vi "Smart_Traffic_Light_System_Main.vi"() -> ()   [LabVIEW 2022 SP3]
uses:
  Chamath Labview/TrafficLightStates.ctl
  <vilib>/DAQmx/read.llb/DAQmx Read (Analog 1D DBL NChan 1Samp).vi
  <vilib>/DAQmx/write.llb/DAQmx Write (Digital Bool 1Line 1Point).vi
  <vilib>/DAQmx/read.llb/DAQmx Read (Digital Bool 1Line 1Point).vi
  <vilib>/Utility/error.llb/Trim Whitespace One-Sided.vi
  <vilib>/DAQmx/create/channels.llb/DAQmx Create Channel (DO-Digital Output).vi
  <vilib>/DAQmx/create/channels.llb/DAQmx Create Channel (AI-Voltage-Basic).vi
  <vilib>/DAQmx/create/channels.llb/DAQmx Create Channel (DI-Digital Input).vi
  <vilib>/DAQmx/miscellaneous.llb/DAQmx Fill In Error Info.vi
panel:
  out "?":string
  out "Street Lights":bool
  in  "Rain signal":tag
  out "Temp 2":bool
  out "Temp 1":bool
  in  "Ped Green":tag
  in  "Ped red":tag
  in  "Numeric":dbl
  out "Square 2":dynamicdata(graph) caption="Square"
  in  "Amplitude":dbl=2.5
  in  "Offset":dbl=2.5
  in  "Frequency":dbl=50.0
  in  "stop (F)":bool
  out "Heavy Rain":bool
  out "Stop Light":bool
  out "Level 7":bool
  out "?":string
  out "Medium rain":bool
  out "Light rain":bool
  out "No rain":bool
  out "?":string
  out "Level 6":bool
  out "Level 5":bool
  out "Level 4":bool
  out "Level 3":bool
  out "Level 2":bool
  out "Level 1":bool
  out "?":string
  out "?":string
  in  "?":bool
  out "?":string
  out "?":string
  in  "Heavy Rain threshold":dbl
  in  "LDR Threshold":dbl
  in  "Buzzer 2":u16(ring) items=["DO0", "DO1", "DO4", "DO5", "DO6"]
  in  "LDR 2":u16(ring) items=["AI1", "AI2", "AI3", "AI4"]
  in  "Rain sensor":u16(ring) items=["AI1", "AI1", "AI3", "AI4"]
  out "Pedestrian in":bool
  out "Push Switch In":bool
  in  "push switch":tag
  out "Push Switch":bool
  out "Rain":bool
  in  "Rain Sensor Output Channel":tag
  in  "LDR output channel":tag
  out "LDR voltage":dbl(knob) scale=0.0..5.0
  out "Rain Sensor Voltage":dbl(knob) scale=0.0..10.0
  in  "Analog input channel":tag
  in  "buzzer - Po.0":tag
  out "Buzzer":bool
  out "RED":bool
  out "YELLOW":bool
  out "green":bool
  out "Pedestrians":bool
  in  "DAQmx Physical Channel 6":tag
  in  "DAQmx Physical Channel 5":tag
  in  "DAQmx Physical Channel 4":tag
  in  "Enum":T1
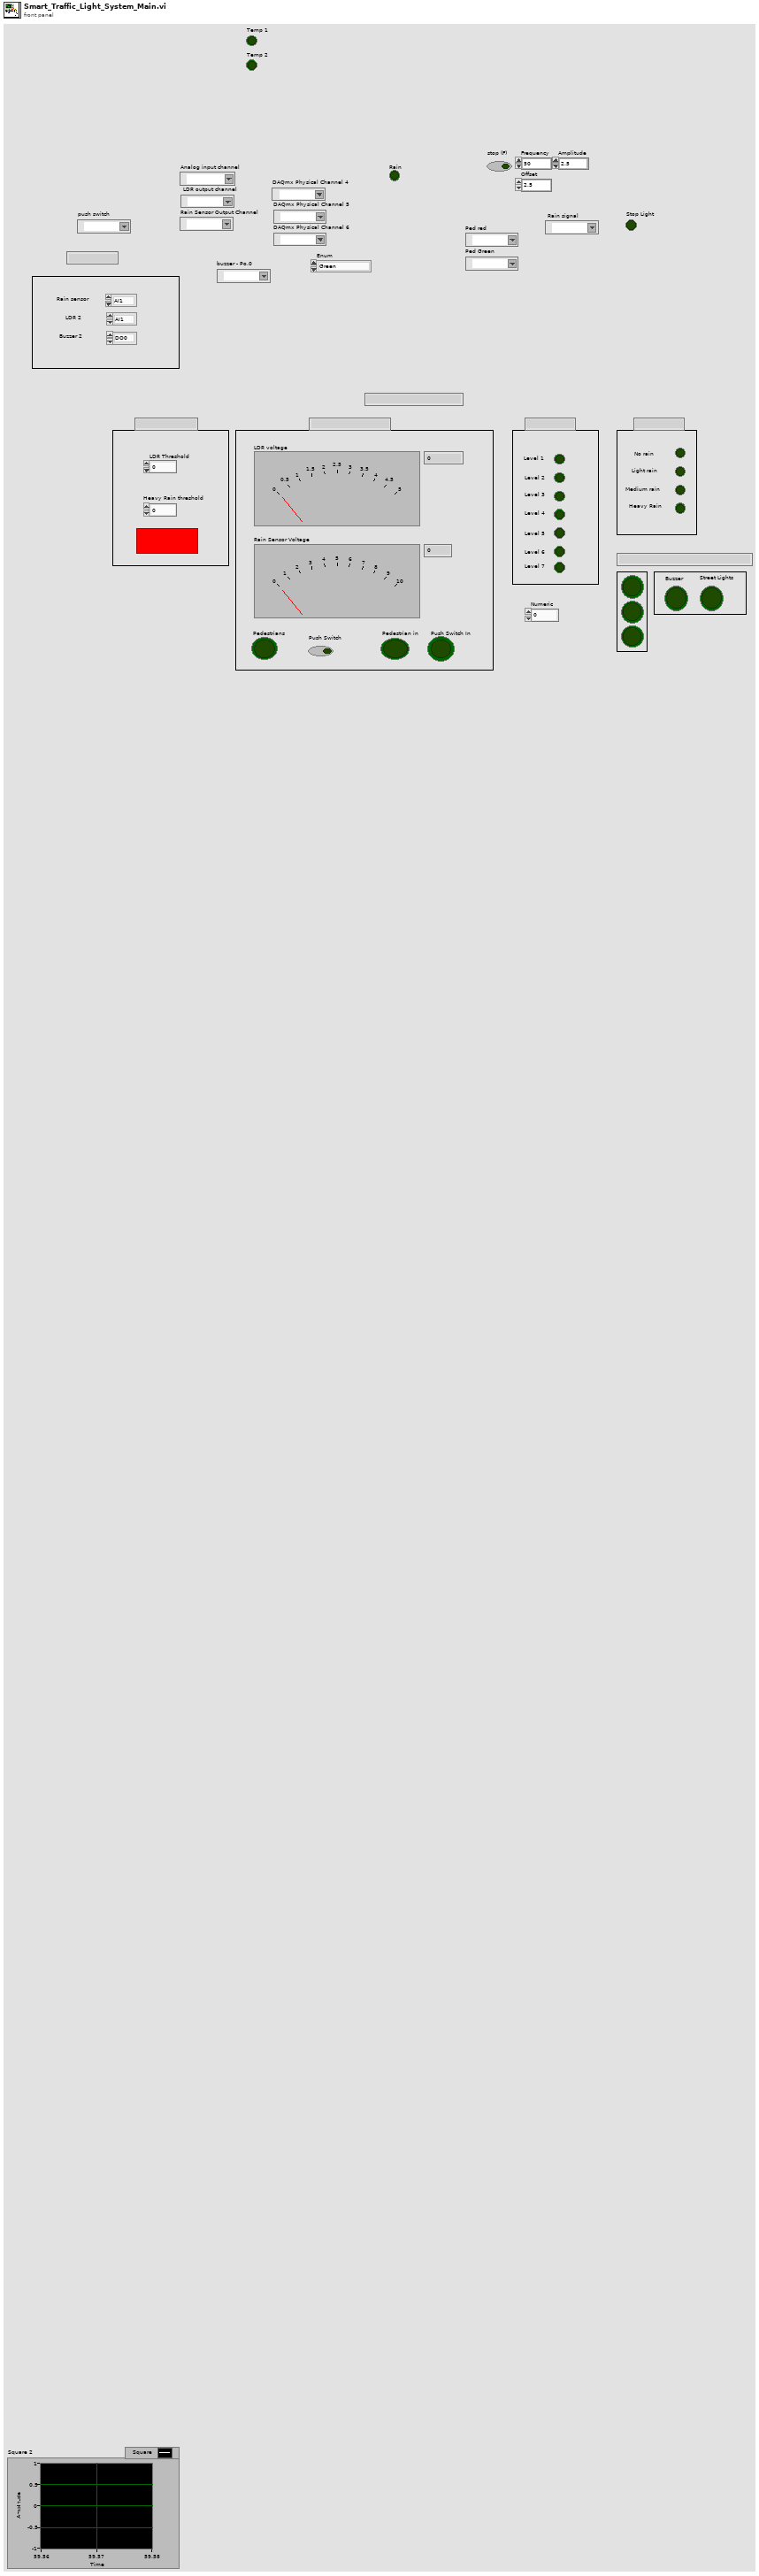
[diagram p1: front panel]
types:
  T1 = typedef "TrafficLightStates.ctl" = enum16{"Green", "Yellow1", "Red", "Yellow2"}
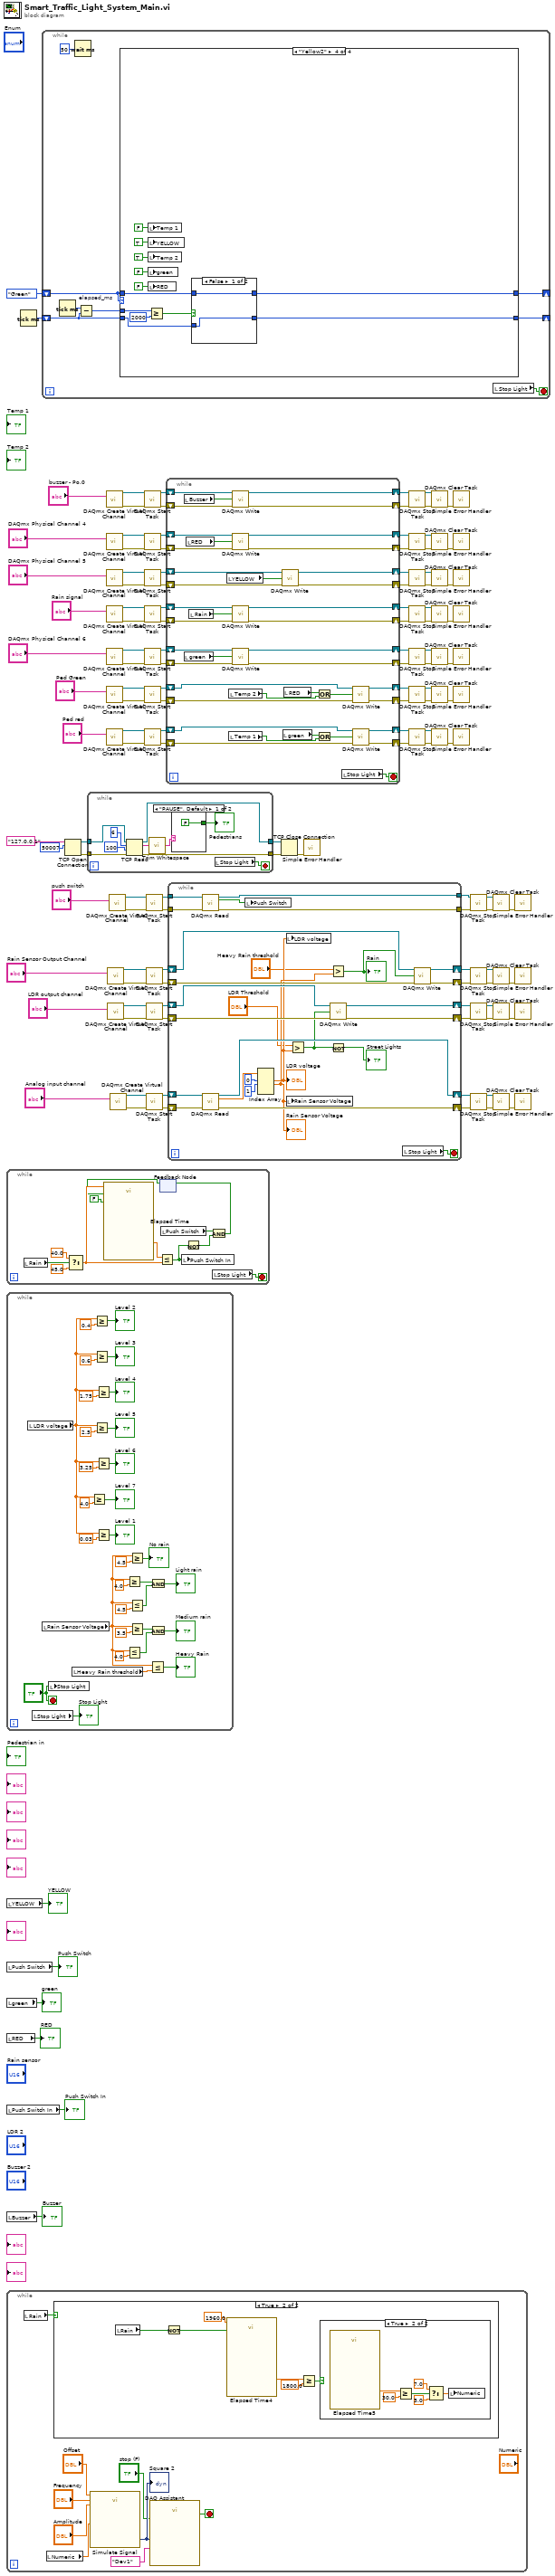
[diagram p0: block diagram]
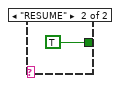
[diagram p4: hidden frame]
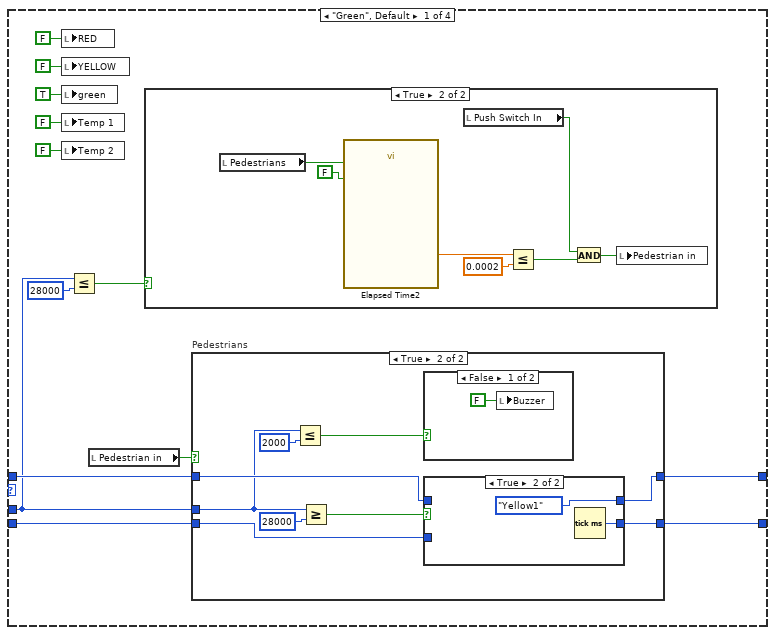
[diagram p5: hidden frame]
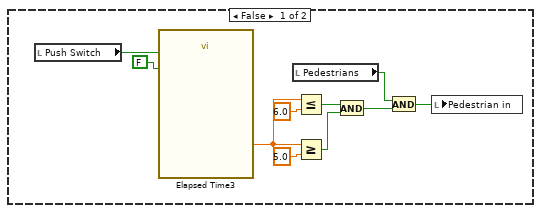
[diagram p6: hidden frame]
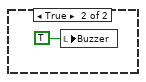
[diagram p8: hidden frame]
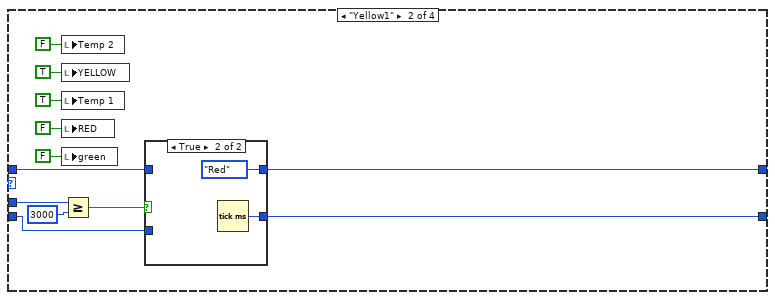
[diagram p10: hidden frame]
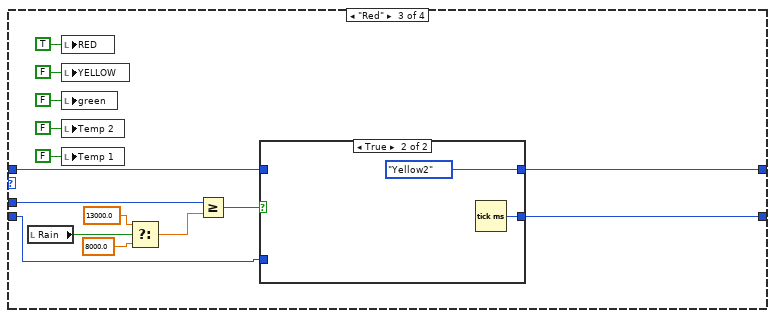
[diagram p12: hidden frame]
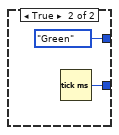
[diagram p14: hidden frame]
diagram:
  n1 = while {
    stop <- w126 stop-if-true
    n2 = local read "Rain"() -> (w135:bool)
    n3 = Select(t=40.0, s=w135, f=45.0) -> (s? t:f=w132:dbl)
    n4 = feedback #1() -> (w127:bool)  [unwired: 1 in]
    n5 = call "Elapsed Time"("Time Target (s)"=w132, "Reset"=w127, "Auto Reset"=FALSE) -> ("Elapsed Time (s)"=w136:dbl)  [unwired: 9 in, 7 out]
    n6 = Less Or Equal?(x=w136, y=w132) -> (x <= y?=w130:bool)
    n7 = local read "Push Switch"() -> (w131:bool)
    n8 = local write "Push Switch In"(w130) -> ()
    n9 = Not(x=w130) -> (.not. x?=w129:bool)
    n10 = And(x=w131, y=w129) -> (x .and. y?=w128:bool)
    n11 = feedback-in #1(w128) -> ()
    n12 = local read "Stop Light"() -> (w126:bool)
  }
  n13 = while {
    stop <- "?" stop-if-true
    n14 = local read "LDR voltage"() -> (w167:dbl)
    n15 = local read "Stop Light"() -> (→"Stop Light":bool)
    n16 = local read "Rain Sensor Voltage"() -> (w152:dbl)
    n17 = local write "Stop Light"("?") -> ()
    n18 = local read "Heavy Rain threshold"() -> (w138:dbl)
    n19 = Greater Or Equal?(x=w167, y=4.0) -> (x >= y?=→"Level 7":bool)
    n20 = Greater Or Equal?(x=w167, y=0.4) -> (x >= y?=→"Level 2":bool)
    n21 = Greater Or Equal?(x=w167, y=0.6) -> (x >= y?=→"Level 3":bool)
    n22 = Greater Or Equal?(x=w167, y=2.5) -> (x >= y?=→"Level 5":bool)
    n23 = Greater Or Equal?(x=w167, y=1.75) -> (x >= y?=→"Level 4":bool)
    n24 = Greater Or Equal?(x=w167, y=3.25) -> (x >= y?=→"Level 6":bool)
    n25 = Greater Or Equal?(x=w167, y=0.03) -> (x >= y?=→"Level 1":bool)
    n26 = Greater Or Equal?(x=w152, y=4.0) -> (x >= y?=w146:bool)
    n27 = Less Or Equal?(x=w152, y=4.0) -> (x <= y?=w143:bool)
    n28 = Greater Or Equal?(x=w152, y=4.5) -> (x >= y?=→"No rain":bool)
    n29 = Less Or Equal?(x=w152, y=4.5) -> (x <= y?=w145:bool)
    n30 = Greater Or Equal?(x=w152, y=3.5) -> (x >= y?=w144:bool)
    n31 = Less Or Equal?(x=w152, y=w138) -> (x <= y?=→"Heavy Rain":bool)
    n32 = And(x=w146, y=w145) -> (x .and. y?=→"Light rain":bool)
    n33 = And(x=w144, y=w143) -> (x .and. y?=→"Medium rain":bool)
  }
  n34 = local read "YELLOW"() -> (→"YELLOW":bool)
  n35 = local read "Push Switch"() -> (→"Push Switch":bool)
  n36 = local read "green"() -> (→"green":bool)
  n37 = local read "RED"() -> (→"RED":bool)
  n38 = local read "Push Switch In"() -> (→"Push Switch In":bool)
  n39 = local read "Buzzer"() -> (→"Buzzer":bool)
  n40 = while {
    stop <- w178 stop-if-true
    n41 = local read "Rain"() -> (w171:bool)
    n42 = local read "Numeric"() -> (w170:dbl)
    n43 = case shown="True" w171 {
      frame False {
      }
      frame True {
        n44 = local read "Rain"() -> (w183:bool)
        n45 = Not(x=w183) -> (.not. x?=w182:bool)
        n46 = call "Elapsed Time4"("Time Target (s)"=1960.0, "Reset"=w182) -> ("Elapsed Time (s)"=w181:dbl)  [unwired: 10 in, 7 out]
        n47 = Greater Or Equal?(x=w181, y=1800.0) -> (x >= y?=w179:bool)
        n48 = case shown="True" w179 {
          frame False {
          }
          frame True {
            n49 = call "Elapsed Time5"() -> ("Elapsed Time (s)"=w190:dbl)  [unwired: 12 in, 7 out]
            n50 = Greater Or Equal?(x=w190, y=30.0) -> (x >= y?=w188:bool)
            n51 = Select(t=7.0, s=w188, f=3.0) -> (s? t:f=w185:dbl)
            n52 = local write "Numeric"(w185) -> ()
          }
        }
      }
    }
    n53 = call "Simulate Signal"("Offset"="Offset", "Duty Cycle (%)"=w170, "Frequency"="Frequency", "Amplitude"="Amplitude") -> ("Square"=w177:dynamicdata)  [unwired: 10 in, 1 out]
    "Square 2" <- w177
    n54 = call "DAQ Assistant"("data"=w177, "stop (F)"="stop (F)", "device name"=tag "Dev1") -> ("stopped"=w178:bool)  [unwired: 14 in, 2 out]
  }
  n55 = Tick Count (ms)() -> (millisecond timer value=w125:u32)
  n56 = while {
    shift-right: [w196] -> _
    shift-left: TrafficLightStates."Green" ("Enum") -> [w197]
    shift-right: [w194] -> _
    shift-left: w125 -> [w195]
    stop <- w191 stop-if-true
    n57 = Tick Count (ms)() -> (millisecond timer value=w198:u32)
    n58 = Wait (ms)(milliseconds to wait=u32 50) -> ()  [unwired: 1 out]
    n59 = Subtract "elapsed_ms"(x=w198, y=w195) -> (x-y=w193:u32)
    n60 = case shown="\"Yellow2\"" w197 {
      tunnel: w197 -> [w211 w252 w271 w287]
      tunnel: [w210 w254 w272 w289] -> w196
      tunnel: w195 -> [w209 w251 w270 w286]
      tunnel: [w208 w253 w269 w288] -> w194
      tunnel: w193 -> [w204 w257 w274 w292]
      frame "Green", Default {
        n61 = local write "RED"(FALSE ("red")) -> ()
        n62 = local write "YELLOW"(FALSE ("yellow")) -> ()
        n63 = local write "green"(TRUE ("green")) -> ()
        n64 = local write "Temp 1"(FALSE ("Temp 1")) -> ()
        n65 = local write "Temp 2"(FALSE ("Temp 2")) -> ()
        n66 = Less Or Equal?(x=w204, y=u32 28000) -> (x <= y?=w202:bool)
        n67 = local read "Pedestrian in"() -> (w201:bool)
        n68 = case shown="True" w202 {
          frame False {
            n69 = local read "Push Switch"() -> (w221:bool)
            n70 = call "Elapsed Time3"("Reset"=w221, "Auto Reset"=FALSE) -> ("Elapsed Time (s)"=w219:dbl)  [unwired: 10 in, 7 out]
            n71 = local read "Pedestrians"() -> (w214:bool)
            n72 = Less Or Equal?(x=w219, y=6.0) -> (x <= y?=w216:bool)
            n73 = Greater Or Equal?(x=w219, y=5.0) -> (x >= y?=w215:bool)
            n74 = And(x=w216, y=w215) -> (x .and. y?=w213:bool)
            n75 = And(x=w214, y=w213) -> (x .and. y?=w212:bool)
            n76 = local write "Pedestrian in"(w212) -> ()
          }
          frame True {
            n77 = local read "Pedestrians"() -> (w228:bool)
            n78 = call "Elapsed Time2"("Reset"=w228, "Auto Reset"=FALSE) -> ("Elapsed Time (s)"=w226:dbl)  [unwired: 10 in, 7 out]
            n79 = local read "Push Switch In"() -> (w224:bool)
            n80 = Less Or Equal?(x=w226, y=0.0002) -> (x <= y?=w223:bool)
            n81 = And(x=w224, y=w223) -> (x .and. y?=w222:bool)
            n82 = local write "Pedestrian in"(w222) -> ()
          }
        }
        n83 = case "Pedestrians" shown="True" w201 {
          tunnel: w211 -> [w230 w235]
          tunnel: [w230 w237] -> w210
          tunnel: w209 -> [w229 w234]
          tunnel: [w229 w236] -> w208
          tunnel: w204 -> [_ w233]
          frame False {
          }
          frame True {
            n84 = Less Or Equal?(x=w233, y=u32 2000) -> (x <= y?=w231:bool)
            n85 = Greater Or Equal?(x=w233, y=u32 28000) -> (x >= y?=w238:bool)
            n86 = case shown="False" w231 {
              frame False {
                n87 = local write "Buzzer"(FALSE ("Buzzer")) -> ()
              }
              frame True {
                n88 = local write "Buzzer"(TRUE ("Buzzer")) -> ()
              }
            }
            n89 = case shown="True" w238 {
              tunnel: [w243 TrafficLightStates."Yellow1" ("Enum")] -> w237
              tunnel: [w242 w244] -> w236
              tunnel: w235 -> [w243 _]
              tunnel: w234 -> [w242 _]
              frame False {
              }
              frame True {
                n90 = Tick Count (ms)() -> (millisecond timer value=w244:u32)
              }
            }
          }
        }
      }
      frame "Yellow1" {
        n91 = local write "Temp 2"(FALSE ("Temp 2")) -> ()
        n92 = local write "YELLOW"(TRUE ("yellow")) -> ()
        n93 = local write "Temp 1"(TRUE ("Temp 1")) -> ()
        n94 = local write "RED"(FALSE ("red")) -> ()
        n95 = local write "green"(FALSE ("green")) -> ()
        n96 = Greater Or Equal?(x=w257, y=u32 3000) -> (x >= y?=w255:bool)
        n97 = case shown="True" w255 {
          tunnel: [w259 TrafficLightStates."Red" ("Enum")] -> w254
          tunnel: [w258 w260] -> w253
          tunnel: w252 -> [w259 _]
          tunnel: w251 -> [w258 _]
          frame False {
          }
          frame True {
            n98 = Tick Count (ms)() -> (millisecond timer value=w260:u32)
          }
        }
      }
      frame "Red" {
        n99 = local read "Rain"() -> (w264:bool)
        n100 = local write "RED"(TRUE ("red")) -> ()
        n101 = local write "YELLOW"(FALSE ("yellow")) -> ()
        n102 = local write "green"(FALSE ("green")) -> ()
        n103 = local write "Temp 2"(FALSE ("Temp 2")) -> ()
        n104 = local write "Temp 1"(FALSE ("Temp 1")) -> ()
        n105 = Select(t=13000.0, s=w264, f=8000.0) -> (s? t:f=w268:dbl)
        n106 = Greater Or Equal?(x=w274, y=w268) -> (x >= y?=w273:bool)
        n107 = case shown="True" w273 {
          tunnel: [w278 TrafficLightStates."Yellow2" ("Enum")] -> w272
          tunnel: w271 -> [w278 _]
          tunnel: [w277 w279] -> w269
          tunnel: w270 -> [w277 _]
          frame False {
          }
          frame True {
            n108 = Tick Count (ms)() -> (millisecond timer value=w279:u32)
          }
        }
      }
      frame "Yellow2" {
        n109 = local write "Temp 1"(FALSE ("Temp 1")) -> ()
        n110 = local write "YELLOW"(TRUE ("yellow")) -> ()
        n111 = local write "Temp 2"(TRUE ("Temp 2")) -> ()
        n112 = local write "green"(FALSE ("green")) -> ()
        n113 = local write "RED"(FALSE ("red")) -> ()
        n114 = Greater Or Equal?(x=w292, y=u32 2000) -> (x >= y?=w290:bool)
        n115 = case shown="False" w290 {
          tunnel: [w294 TrafficLightStates."Green" ("Enum")] -> w289
          tunnel: [w293 w295] -> w288
          tunnel: w287 -> [w294 _]
          tunnel: w286 -> [w293 _]
          frame False {
          }
          frame True {
            n116 = Tick Count (ms)() -> (millisecond timer value=w295:u32)
          }
        }
      }
    }
    n117 = local read "Stop Light"() -> (w191:bool)
  }
  n118 = TCP Open Connection(address="127.0.0.1", remote port or service name=u16 50007) -> (connection ID=w90:refnum<k5>, error out=w91:errorcluster)  [unwired: 3 in]
  n119 = while {
    tunnel: [w302] -> w92
    tunnel: w91 -> [w301]
    tunnel: w90 -> [w300]
    tunnel: [w299] -> w89
    stop <- w297 stop-if-true
    n120 = TCP Read(connection ID=w300, bytes to read=6, error in (no error)=w301, 9:100 ("timeout ms (25000)")) -> (connection ID out=w302:refnum<k5>, data out=w304:string, error out=w299:errorcluster)  [unwired: 1 in]
    n121 = call <vilib>:"Trim Whitespace.vi"("string"=w304) -> ("trimmed string"=w303:string)  [unwired: 1 in]
    n122 = case shown="\"PAUSE\", Default" w303 {
      tunnel: [FALSE TRUE] -> w298
      frame "PAUSE", Default {
      }
      frame "RESUME" {
      }
    }
    "Pedestrians" <- w298
    n123 = local read "Stop Light"() -> (w297:bool)
  }
  n124 = call-poly <vilib>:"DAQmx Create Virtual Channel.vi"("lines"="buzzer - Po.0") -> ("task out"=w85:refnum<k21>, "error out"=w84:errorcluster)  [unwired: 13 in]
  n125 = call-poly <vilib>:"DAQmx Create Virtual Channel.vi"("lines"="DAQmx Physical Channel 4") -> ("task out"=w123:refnum<k21>, "error out"=w122:errorcluster)  [unwired: 13 in]
  n126 = call-poly <vilib>:"DAQmx Create Virtual Channel.vi"("lines"="DAQmx Physical Channel 5") -> ("task out"=w117:refnum<k21>, "error out"=w116:errorcluster)  [unwired: 13 in]
  n127 = call-poly <vilib>:"DAQmx Create Virtual Channel.vi"("lines"="Rain signal") -> ("task out"=w9:refnum<k21>, "error out"=w8:errorcluster)  [unwired: 13 in]
  n128 = call-poly <vilib>:"DAQmx Create Virtual Channel.vi"("lines"="DAQmx Physical Channel 6") -> ("task out"=w111:refnum<k21>, "error out"=w110:errorcluster)  [unwired: 13 in]
  n129 = call-poly <vilib>:"DAQmx Create Virtual Channel.vi"("lines"="Ped Green") -> ("task out"=w26:refnum<k21>, "error out"=w25:errorcluster)  [unwired: 13 in]
  n130 = call-poly <vilib>:"DAQmx Create Virtual Channel.vi"("lines"="Ped red") -> ("task out"=w29:refnum<k21>, "error out"=w28:errorcluster)  [unwired: 13 in]
  n131 = call-poly <vilib>:"DAQmx Create Virtual Channel.vi"("lines"="Rain Sensor Output Channel") -> ("task out"=w55:refnum<k21>, "error out"=w54:errorcluster)  [unwired: 13 in]
  n132 = call-poly <vilib>:"DAQmx Create Virtual Channel.vi"("lines"="LDR output channel") -> ("task out"=w64:refnum<k21>, "error out"=w63:errorcluster)  [unwired: 13 in]
  n133 = call-poly <vilib>:"DAQmx Create Virtual Channel.vi"("lines"="push switch") -> ("task out"=w44:refnum<k21>, "error out"=w43:errorcluster)  [unwired: 13 in]
  n134 = call-poly <vilib>:"DAQmx Create Virtual Channel.vi"("physical channels"="Analog input channel") -> ("task out"=w74:refnum<k21>, "error out"=w73:errorcluster)  [unwired: 13 in]
  n135 = call <vilib>:"DAQmx Start Task.vi"("task/channels in"=w85, "error in"=w84) -> ("task out"=w83:refnum<k21>, "error out"=w82:errorcluster)  [unwired: 12 in]
  n136 = call <vilib>:"DAQmx Start Task.vi"("task/channels in"=w123, "error in"=w122) -> ("task out"=w98:refnum<k21>, "error out"=w96:errorcluster)  [unwired: 12 in]
  n137 = call <vilib>:"DAQmx Start Task.vi"("task/channels in"=w117, "error in"=w116) -> ("task out"=w102:refnum<k21>, "error out"=w101:errorcluster)  [unwired: 12 in]
  n138 = call <vilib>:"DAQmx Start Task.vi"("task/channels in"=w9, "error in"=w8) -> ("task out"=w4:refnum<k21>, "error out"=w2:errorcluster)  [unwired: 12 in]
  n139 = call <vilib>:"DAQmx Start Task.vi"("task/channels in"=w111, "error in"=w110) -> ("task out"=w106:refnum<k21>, "error out"=w105:errorcluster)  [unwired: 12 in]
  n140 = call <vilib>:"DAQmx Start Task.vi"("task/channels in"=w26, "error in"=w25) -> ("task out"=w16:refnum<k21>, "error out"=w15:errorcluster)  [unwired: 12 in]
  n141 = call <vilib>:"DAQmx Start Task.vi"("task/channels in"=w29, "error in"=w28) -> ("task out"=w18:refnum<k21>, "error out"=w17:errorcluster)  [unwired: 12 in]
  n142 = call <vilib>:"DAQmx Start Task.vi"("task/channels in"=w44, "error in"=w43) -> ("task out"=w39:refnum<k21>, "error out"=w38:errorcluster)  [unwired: 12 in]
  n143 = call <vilib>:"DAQmx Start Task.vi"("task/channels in"=w55, "error in"=w54) -> ("task out"=w52:refnum<k21>, "error out"=w51:errorcluster)  [unwired: 12 in]
  n144 = call <vilib>:"DAQmx Start Task.vi"("task/channels in"=w64, "error in"=w63) -> ("task out"=w62:refnum<k21>, "error out"=w61:errorcluster)  [unwired: 12 in]
  n145 = call <vilib>:"DAQmx Start Task.vi"("task/channels in"=w74, "error in"=w73) -> ("task out"=w72:refnum<k21>, "error out"=w71:errorcluster)  [unwired: 12 in]
  n146 = while {
    shift-right: [w346] -> w104
    shift-left: w106 -> [w348]
    shift-right: [w345] -> w103
    shift-left: w105 -> [w347]
    shift-right: [w342] -> w100
    shift-left: w102 -> [w344]
    shift-right: [w341] -> w99
    shift-left: w101 -> [w343]
    shift-right: [w339] -> w97
    shift-left: w98 -> [w340]
    shift-right: [w337] -> w95
    shift-left: w96 -> [w338]
    shift-right: [w331] -> w81
    shift-left: w83 -> [w333]
    shift-right: [w330] -> w80
    shift-left: w82 -> [w332]
    shift-right: [w321] -> w12
    shift-left: w16 -> [w325]
    shift-right: [w320] -> w11
    shift-left: w15 -> [w324]
    shift-right: [w323] -> w14
    shift-left: w18 -> [w327]
    shift-right: [w322] -> w13
    shift-left: w17 -> [w326]
    shift-right: [w312] -> w3
    shift-left: w4 -> [w313]
    shift-right: [w310] -> w1
    shift-left: w2 -> [w311]
    stop <- w328 stop-if-true
    n147 = local read "Buzzer"() -> (w329:bool)
    n148 = local read "green"() -> (w336:bool)
    n149 = local read "RED"() -> (w334:bool)
    n150 = local read "Rain"() -> (w309:bool)
    n151 = local read "YELLOW"() -> (w335:bool)
    n152 = local read "Temp 2"() -> (w317:bool)
    n153 = local read "Temp 1"() -> (w316:bool)
    n154 = call-poly <vilib>:"DAQmx Write.vi"("task/channels in"=w333, "data"=w329, "error in"=w332) -> ("task out"=w331:refnum<k21>, "error out"=w330:errorcluster)  [unwired: 10 in, 1 out]
    n155 = call-poly <vilib>:"DAQmx Write.vi"("task/channels in"=w340, "data"=w334, "error in"=w338) -> ("task out"=w339:refnum<k21>, "error out"=w337:errorcluster)  [unwired: 10 in, 1 out]
    n156 = call-poly <vilib>:"DAQmx Write.vi"("task/channels in"=w313, "data"=w309, "error in"=w311) -> ("task out"=w312:refnum<k21>, "error out"=w310:errorcluster)  [unwired: 10 in, 1 out]
    n157 = call-poly <vilib>:"DAQmx Write.vi"("task/channels in"=w348, "data"=w336, "error in"=w347) -> ("task out"=w346:refnum<k21>, "error out"=w345:errorcluster)  [unwired: 10 in, 1 out]
    n158 = call-poly <vilib>:"DAQmx Write.vi"("task/channels in"=w344, "data"=w335, "error in"=w343) -> ("task out"=w342:refnum<k21>, "error out"=w341:errorcluster)  [unwired: 10 in, 1 out]
    n159 = local read "green"() -> (w318:bool)
    n160 = local read "RED"() -> (w319:bool)
    n161 = Or(x=w319, y=w317) -> (x .or. y?=w314:bool)
    n162 = Or(x=w318, y=w316) -> (x .or. y?=w315:bool)
    n163 = local read "Stop Light"() -> (w328:bool)
    n164 = call-poly <vilib>:"DAQmx Write.vi"("task/channels in"=w325, "data"=w314, "error in"=w324) -> ("task out"=w321:refnum<k21>, "error out"=w320:errorcluster)  [unwired: 10 in, 1 out]
    n165 = call-poly <vilib>:"DAQmx Write.vi"("task/channels in"=w327, "data"=w315, "error in"=w326) -> ("task out"=w323:refnum<k21>, "error out"=w322:errorcluster)  [unwired: 10 in, 1 out]
  }
  n166 = while {
    shift-right: [w374] -> w70
    shift-left: w72 -> [w376]
    shift-right: [w373] -> w69
    shift-left: w71 -> [w375]
    shift-right: [w370] -> w60
    shift-left: w62 -> [w372]
    shift-right: [w369] -> w59
    shift-left: w61 -> [w371]
    shift-right: [w362] -> w47
    shift-left: w52 -> [w365]
    shift-right: [w363] -> w46
    shift-left: w51 -> [w364]
    tunnel: w39 -> [w360]
    tunnel: w38 -> [w359]
    tunnel: [w358] -> w37
    tunnel: [w357] -> w36
    stop <- w351 stop-if-true
    n167 = call-poly <vilib>:"DAQmx Read.vi"("task/channels in"=w360, "error in"=w359) -> ("task out"=w358:refnum<k21>, "data"=w356:bool, "error out"=w357:errorcluster)  [unwired: 11 in]
    n168 = call-poly <vilib>:"DAQmx Read.vi"("task/channels in"=w376, "error in"=w375) -> ("task out"=w374:refnum<k21>, "data"=w368:dbl[], "error out"=w373:errorcluster)  [unwired: 11 in]
    n169 = local write "Push Switch"(w356) -> ()
    n170 = Index Array(array=w368, index #1=0 ("index"), index #2=1 ("index")) -> (element #1=w354:dbl, element #2=w355:dbl)  [unwired: 2 in, 2 out]
    "LDR voltage" <- w354
    "Rain Sensor Voltage" <- w355
    n171 = local write "LDR voltage"(w354) -> ()
    n172 = local write "Rain Sensor Voltage"(w355) -> ()
    n173 = Greater?(x="LDR Threshold", y=w354) -> (0:w350:bool)
    n174 = Greater?(x="Heavy Rain threshold", y=w355) -> (0:w361:bool)
    "Rain" <- w361
    n175 = call-poly <vilib>:"DAQmx Write.vi"("task/channels in"=w372, "data"=w350, "error in"=w371) -> ("task out"=w370:refnum<k21>, "error out"=w369:errorcluster)  [unwired: 10 in, 1 out]
    n176 = Not(x=w350) -> (.not. x?=→"Street Lights":bool)
    n177 = local read "Stop Light"() -> (w351:bool)
    n178 = call-poly <vilib>:"DAQmx Write.vi"("task/channels in"=w365, "data"=w361, "error in"=w364) -> ("task out"=w362:refnum<k21>, "error out"=w363:errorcluster)  [unwired: 10 in, 1 out]
  }
  n179 = TCP Close Connection(connection ID=w92, error in (no error)=w89) -> (error out=w88:errorcluster)  [unwired: 1 in, 1 out]
  n180 = call <vilib>:"Simple Error Handler.vi"("error in (no error)"=w88) -> ()  [unwired: 4 in, 5 out]
  n181 = call <vilib>:"DAQmx Stop Task.vi"("task/channels in"=w81, "error in"=w80) -> ("task out"=w79:refnum<k21>, "error out"=w78:errorcluster)  [unwired: 12 in]
  n182 = call <vilib>:"DAQmx Stop Task.vi"("task/channels in"=w97, "error in"=w95) -> ("task out"=w121:refnum<k21>, "error out"=w120:errorcluster)  [unwired: 12 in]
  n183 = call <vilib>:"DAQmx Stop Task.vi"("task/channels in"=w100, "error in"=w99) -> ("task out"=w115:refnum<k21>, "error out"=w114:errorcluster)  [unwired: 12 in]
  n184 = call <vilib>:"DAQmx Stop Task.vi"("task/channels in"=w3, "error in"=w1) -> ("task out"=w7:refnum<k21>, "error out"=w6:errorcluster)  [unwired: 12 in]
  n185 = call <vilib>:"DAQmx Stop Task.vi"("task/channels in"=w104, "error in"=w103) -> ("task out"=w109:refnum<k21>, "error out"=w108:errorcluster)  [unwired: 12 in]
  n186 = call <vilib>:"DAQmx Stop Task.vi"("task/channels in"=w12, "error in"=w11) -> ("task out"=w21:refnum<k21>, "error out"=w20:errorcluster)  [unwired: 12 in]
  n187 = call <vilib>:"DAQmx Stop Task.vi"("task/channels in"=w14, "error in"=w13) -> ("task out"=w24:refnum<k21>, "error out"=w23:errorcluster)  [unwired: 12 in]
  n188 = call <vilib>:"DAQmx Clear Task.vi"("task in"=w79, "error in"=w78) -> ("error out"=w77:errorcluster)  [unwired: 13 in]
  n189 = call <vilib>:"DAQmx Clear Task.vi"("task in"=w121, "error in"=w120) -> ("error out"=w119:errorcluster)  [unwired: 13 in]
  n190 = call <vilib>:"DAQmx Clear Task.vi"("task in"=w115, "error in"=w114) -> ("error out"=w113:errorcluster)  [unwired: 13 in]
  n191 = call <vilib>:"DAQmx Clear Task.vi"("task in"=w7, "error in"=w6) -> ("error out"=w5:errorcluster)  [unwired: 13 in]
  n192 = call <vilib>:"DAQmx Clear Task.vi"("task in"=w109, "error in"=w108) -> ("error out"=w107:errorcluster)  [unwired: 13 in]
  n193 = call <vilib>:"DAQmx Clear Task.vi"("task in"=w21, "error in"=w20) -> ("error out"=w19:errorcluster)  [unwired: 13 in]
  n194 = call <vilib>:"DAQmx Clear Task.vi"("task in"=w24, "error in"=w23) -> ("error out"=w22:errorcluster)  [unwired: 13 in]
  n195 = call <vilib>:"Simple Error Handler.vi"("error in (no error)"=w77) -> ()  [unwired: 4 in, 5 out]
  n196 = call <vilib>:"Simple Error Handler.vi"("error in (no error)"=w119) -> ()  [unwired: 4 in, 5 out]
  n197 = call <vilib>:"Simple Error Handler.vi"("error in (no error)"=w113) -> ()  [unwired: 4 in, 5 out]
  n198 = call <vilib>:"Simple Error Handler.vi"("error in (no error)"=w5) -> ()  [unwired: 4 in, 5 out]
  n199 = call <vilib>:"Simple Error Handler.vi"("error in (no error)"=w107) -> ()  [unwired: 4 in, 5 out]
  n200 = call <vilib>:"Simple Error Handler.vi"("error in (no error)"=w19) -> ()  [unwired: 4 in, 5 out]
  n201 = call <vilib>:"Simple Error Handler.vi"("error in (no error)"=w22) -> ()  [unwired: 4 in, 5 out]
  n202 = call <vilib>:"DAQmx Stop Task.vi"("task/channels in"=w37, "error in"=w36) -> ("task out"=w42:refnum<k21>, "error out"=w41:errorcluster)  [unwired: 12 in]
  n203 = call <vilib>:"DAQmx Stop Task.vi"("task/channels in"=w47, "error in"=w46) -> ("task out"=w50:refnum<k21>, "error out"=w49:errorcluster)  [unwired: 12 in]
  n204 = call <vilib>:"DAQmx Stop Task.vi"("task/channels in"=w60, "error in"=w59) -> ("task out"=w58:refnum<k21>, "error out"=w57:errorcluster)  [unwired: 12 in]
  n205 = call <vilib>:"DAQmx Stop Task.vi"("task/channels in"=w70, "error in"=w69) -> ("task out"=w68:refnum<k21>, "error out"=w67:errorcluster)  [unwired: 12 in]
  n206 = call <vilib>:"DAQmx Clear Task.vi"("task in"=w42, "error in"=w41) -> ("error out"=w40:errorcluster)  [unwired: 13 in]
  n207 = call <vilib>:"DAQmx Clear Task.vi"("task in"=w50, "error in"=w49) -> ("error out"=w48:errorcluster)  [unwired: 13 in]
  n208 = call <vilib>:"DAQmx Clear Task.vi"("task in"=w58, "error in"=w57) -> ("error out"=w56:errorcluster)  [unwired: 13 in]
  n209 = call <vilib>:"DAQmx Clear Task.vi"("task in"=w68, "error in"=w67) -> ("error out"=w66:errorcluster)  [unwired: 13 in]
  n210 = call <vilib>:"Simple Error Handler.vi"("error in (no error)"=w40) -> ()  [unwired: 4 in, 5 out]
  n211 = call <vilib>:"Simple Error Handler.vi"("error in (no error)"=w48) -> ()  [unwired: 4 in, 5 out]
  n212 = call <vilib>:"Simple Error Handler.vi"("error in (no error)"=w56) -> ()  [unwired: 4 in, 5 out]
  n213 = call <vilib>:"Simple Error Handler.vi"("error in (no error)"=w66) -> ()  [unwired: 4 in, 5 out]
